vi "labviewFrequencyResponseDemo.vi"() -> ()   [LabVIEW 2020]
uses:
  <vilib>/Simulation/Scripting/Companion Diagram/SimConfigNode/SimParams.ctl
  <vilib>/Simulation/Scripting/Companion Diagram/SimConfigNode/_simSolvers.ctl
  <vilib>/Simulation/Implementation/Shared/SIMSCR Execution Mode.ctl
  <vilib>/Simulation/Param Hierarchy/Typedefs/SIMPH Param Control Actions.ctl
  <vilib>/Simulation/Implementation/Shared/NILVSim_ParamChanged.vi
  <vilib>/Simulation/Implementation/Shared/NILVSim_FinishedLate.vi
  <vilib>/Simulation/Implementation/Shared/NILVSIM_BeginStep.vi
  <vilib>/Simulation/DataSources/Implementation/NILVSim Signal Generator.llb/SIM Signal Generator (scalar).vi
  <vilib>/Simulation/SignalDisplay/Implementation/NILVSim Time Waveform.llb/SIM Time Waveform (scalar).vi
  <vilib>/Simulation/Utility/Implementation/NILVSim Memory.llb/NILVSim Memory (core).vi
  <vilib>/Simulation/ContinuousLinear/Implementation/NILVSim Transfer Function.llb/SIM Transfer Function Distributor (SISO).vi
  <vilib>/Simulation/ContinuousLinear/Implementation/NILVSim Transfer Function.llb/SIM Transfer Function Collector (SISO).vi
  <vilib>/Simulation/SignalDisplay/Implementation/NILVSim Time Waveform.llb/SIM Time Waveform (vector).vi
  <vilib>/Simulation/Implementation/Shared/NILVSim_Manager.vi
  <vilib>/Utility/error.llb/Clear Errors.vi
  <vilib>/Simulation/Implementation/Shared/NILVSim_FinalizeModel.vi
  <vilib>/Simulation/Implementation/Shared/SIM Unbundle Sim Info.vi
  <vilib>/Simulation/Implementation/Shared/SIMSH Read Queue.vi
  <vilib>/Simulation/Implementation/Shared/NILVSim_Initialize.vi
  <vilib>/Simulation/Utility/Implementation/NILVSim Get Time and IsAcceptedStep.vi
  <vilib>/Simulation/Implementation/Shared/NILVSim_GetModelError.vi
  <vilib>/Simulation/Implementation/Shared/SIM Bundle Sim Info.vi
  <vilib>/Simulation/Scripting/Companion Diagram/SimConfigNode/SimDog.xnode
  <vilib>/Simulation/Implementation/XNodeFramework/SimXNode/SimX.xnode
  <vilib>/Simulation/ContinuousLinear/Implementation/NILVSim Transfer Function.llb/SIM Transfer Function (SISO).vi
  <vilib>/Simulation/Implementation/Shared/NI_SIM_Implementation.lvlib
panel:
  out "CSTR Temp (C)":dbl
  out "Fuel Input (dimensionless)":dbl
  out "Reaction heat":dbl
  out "Fuel input (dimensionless) vs time":waveform(dbl)(graph)
  in  "Heater Oscillation Amplitude\n(fraction of baseline power)":dbl=1.0
  in  "Heater Oscillation Freq\n(Hz)":dbl=0.5
  in  "Baseline Heater Power  Fraction":dbl
  out "Temperature (C) vs Time":waveform(dbl)(graph)
  out "Waveform Chart\nOutput":waveform(dbl)[](graph)
  in  "Input Control":dbl(slide) scale=0.0..10.0
  in  "stop While loop":bool
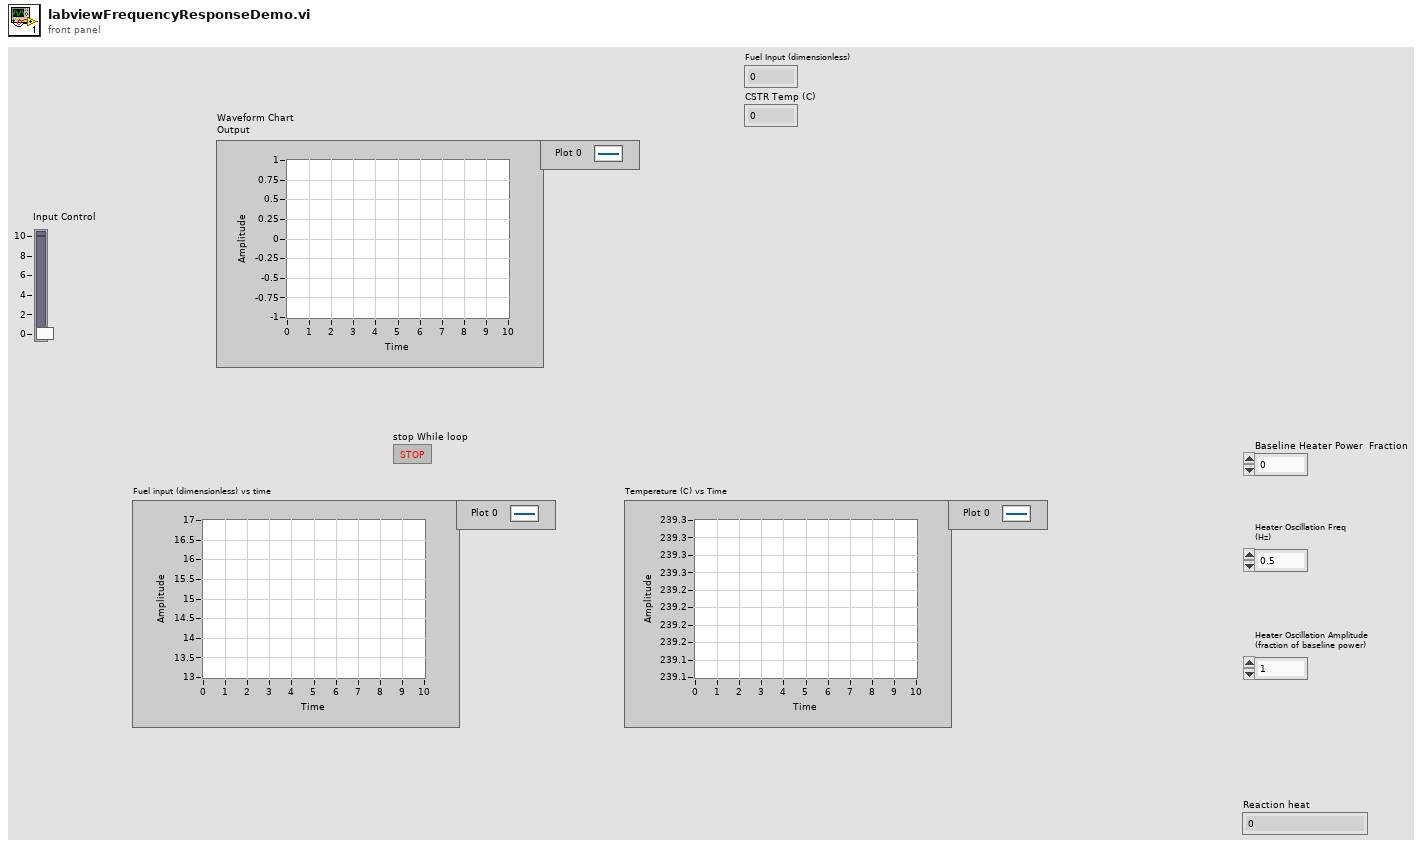
[diagram p1: front panel]
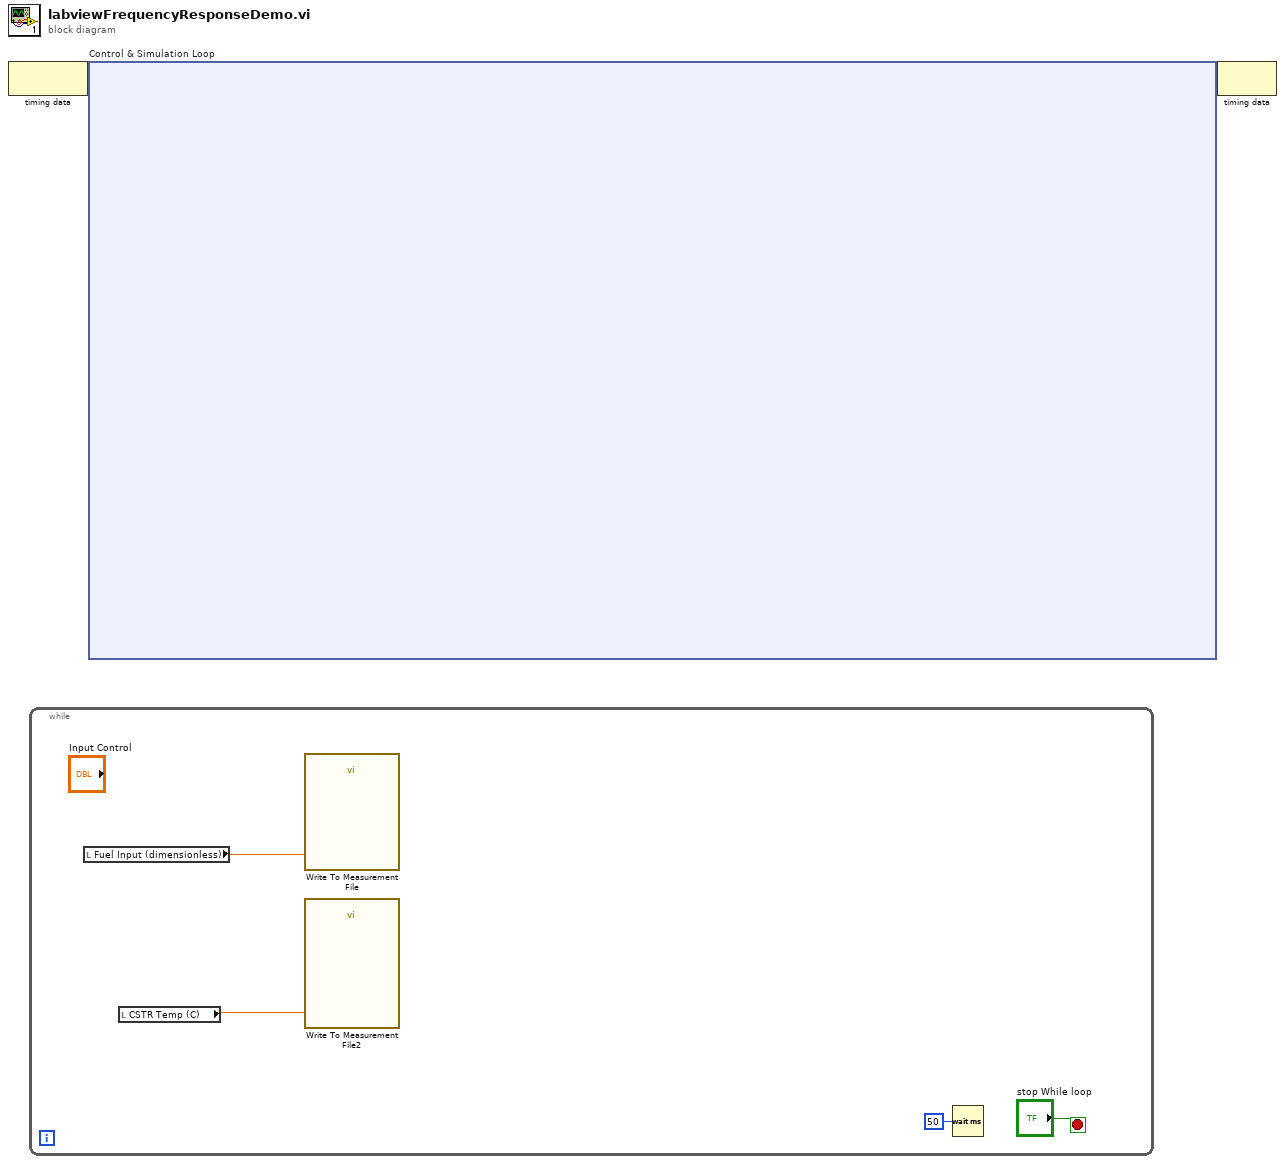
[diagram p0: block diagram]
diagram:
  n1 = node-c288() -> (w2:variant)  [unwired: 1 in]
  n2 = while {
    stop <- "stop While loop" stop-if-true
    n3 = local read "Fuel Input (dimensionless)"() -> (w4:dbl)
    n4 = local read "CSTR Temp (C)"() -> (w3:dbl)
    n5 = call "Write To Measurement File"("Signals"=w4) -> ()  [unwired: 16 in, 3 out]
    n6 = call "Write To Measurement File2"("Signals"=w3) -> ()  [unwired: 16 in, 3 out]
    n7 = Wait (ms)(milliseconds to wait=u32 50) -> ()  [unwired: 1 out]
  }
  n8 = node-c254 "Control & Simulation Loop"(w2) -> (w1:variant)
  n9 = node-c288(w1) -> ()  [unwired: 1 out]
